vi "Read.vi"(8 "error in (no error)":errorcluster, 11 "Two Terminal in":refnum<class "AbsFunc_Two Term_Bool.lvclass">) -> (0 "error out":errorcluster, 2 "Boolean":bool, 3 "Two Terminal out":refnum<class "AbsFunc_Two Term_Bool.lvclass">)   [LabVIEW 2021, in "AbsFunc_Two Term_Bool.lvclass"]
uses:
  AbsFunc_Two Term_Bool.lvclass
  AbsFunc_Two Term_Bool.lvclass/AbsFunc_Two Term_Bool.ctl
  Abs_Types/Boolean/Abs_Boolean.lvclass
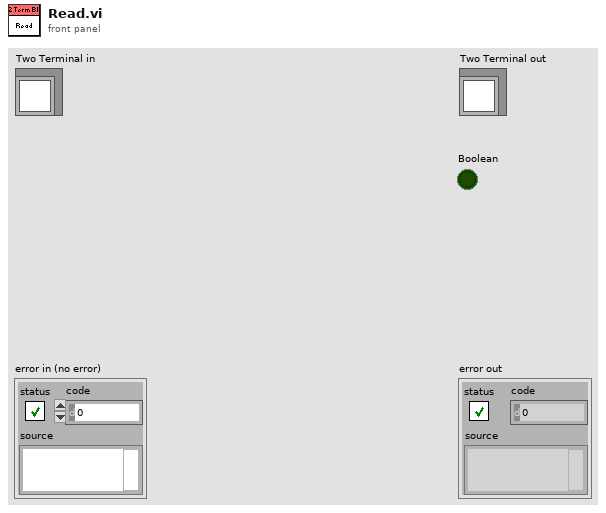
[diagram p1: front panel]
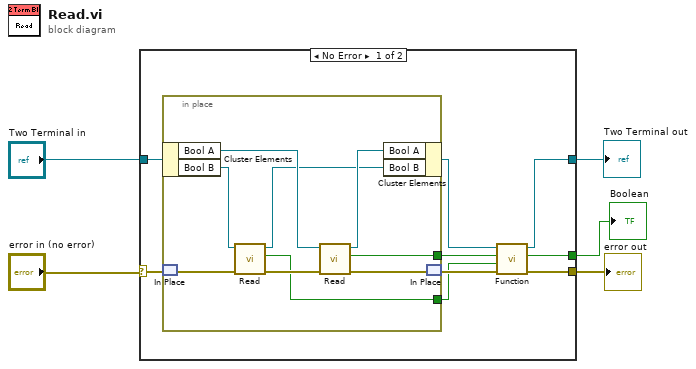
[diagram p0: block diagram]
diagram:
  n1 = case shown="No Error" "error in (no error)" {
    selector: "error in (no error)" -> [w13 w24]
    tunnel: "Two Terminal in" -> [w14 w25]
    tunnel: [w7 w24] -> w3
    tunnel: [w8 w25] -> w2
    tunnel: [w6 _] -> w1
    frame No Error {
      n2 = in-place {
        in-place-border: [w20] -> w10
        in-place-border: [w15] -> w9
        n3 = in-place-cluster #1(w14) -> ("Bool A"=w22:refnum<class "Abs_Boolean.lvclass">, "Bool B"=w17:refnum<class "Abs_Boolean.lvclass">)
        n4 = in-place-match #2(w13) -> (w19:errorcluster)
        n5 = call-dynamic "Read.vi"("error in (no error)"=w19, "Boolean in"=w17) -> ("error out"=w18:errorcluster, "Boolean"=w15:bool, "Boolean out"=w16:refnum<class "Abs_Boolean.lvclass">)  [unwired: 7 in]
        n6 = call-dynamic "Read.vi"("error in (no error)"=w18, "Boolean in"=w22) -> ("error out"=w23:errorcluster, "Boolean"=w20:bool, "Boolean out"=w21:refnum<class "Abs_Boolean.lvclass">)  [unwired: 7 in]
        n7 = in-place-cluster #1("Bool A"=w21, "Bool B"=w16) -> (w12:refnum<class "AbsFunc_Two Term_Bool.lvclass">)
        n8 = in-place-match #2(w23) -> (w11:errorcluster)
      }
      n9 = call-dynamic "Function.vi"("error in (no error)"=w11, "Bool B"=w9, "Bool A"=w10, "Two Terminal in"=w12) -> ("error out"=w7:errorcluster, "Result"=w6:bool, "Two Terminal out"=w8:refnum<class "AbsFunc_Two Term_Bool.lvclass">)  [unwired: 5 in]
    }
    frame Error {
    }
  }
  "error out" <- w3
  "Two Terminal out" <- w2
  "Boolean" <- w1
